vi "IMUBegin.vi"(8 "error in":errorcluster) -> (0 "error out":errorcluster)   [LabVIEW 2014]
uses:
  NavX/roborio/labview/navX-MXP Library/navX-MXP IMU.lvlib
panel:
  out "IMU Opened":bool
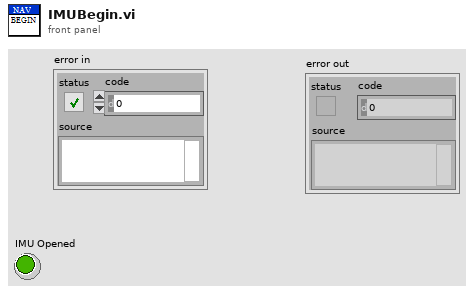
[diagram p1: front panel]
types:
  T1 = typedef "navX-MXP IMU.lvlib/navX Device TypeDef.ctl" = cluster{"navX Interface Protocol":T2, "navX Interface Protocol TypeDefs":cluster{"SPIDevRef":T3, "I2CDevRef":T6}, "navX System Information":cluster{"Board Information":T8, "Status":T9, "Offsets":T13}, "navX Common Information":cluster{"Update Rate (4Hz-60Hz)":T14, "refnum name":string, "error":errorcluster}}
  T2 = typedef "navX-MXP IMU.lvlib/navX Interface Protocol.ctl" = enum16{"SPI", "I2C"}
  T3 = typedef "WPI_SPIDevRef.ctl" = cluster{"DevStatus":errorcluster, "Handle":i32, "Controller":T4, "SPI Bus":T5}
  T4 = typedef "FPGA_TypedefDigitalModule.ctl" = enum16{"Controller 1"}
  T5 = typedef "spi_bus.ctl" = enum16{"SPI On-Board, CS0", "SPI On-Board, CS1", "SPI On-Board, CS2", "SPI On-Board, CS3", "SPI MXP", "Invalid"}
  T6 = typedef "WPI_I2CDevRef.ctl" = cluster{"DevStatus":errorcluster, "Controller":T4, "Device Address":u8, "Handle":i32, "I2C Bus":T7}
  T7 = typedef "i2c_bus.ctl" = enum16{"I2C On-Board", "I2C MXP", "Invalid"}
  T8 = typedef "navX-MXP IMU.lvlib/navX Board Information.ctl" = cluster{"WhoAmI (50 | 0x32)":u8, "Board Revision":u8, "Firmware Major Version":u8, "Firmware Minor Version":u8}
  T9 = typedef "navX-MXP IMU.lvlib/navX Status Data.ctl" = cluster{"Update Rate Hz":u8, "Accelerometer Full-Scale Range":u8, "Gyro Full-Scale Range":u16, "NAVX_OP_STATUS":T10, "NAVX_CAL_STATUS":T11, "NAVX_SELFTEST_STATUS":u8, "NAVX_SENSOR_STATUS":T12}
  T10 = typedef "navX-MXP IMU.lvlib/navX NAVX_OP_STATUS.ctl" = u8
  T11 = typedef "navX-MXP IMU.lvlib/navX NAVX_CAL_STATUS.ctl" = u8
  T12 = typedef "navX-MXP IMU.lvlib/navX NAVX_SENSOR_STATUS.ctl" = cluster{"MOVING":bool, "YAW_STABLE":bool, "MAG_DISTURBANCE":bool, "ALTITUDE_VALID":bool, "SEALEVEL_PRESS_SET":bool, "FUSED_HEADING_VALID":bool}
  T13 = typedef "navX-MXP IMU.lvlib/navX Offsets Data.ctl" = cluster{"Yaw":dbl, "Quat W":dbl, "Quat X":dbl, "Quat Y":dbl, "Quat Z":dbl}
  T14 = typedef "navX-MXP IMU.lvlib/navX Update Rate.ctl" = u8
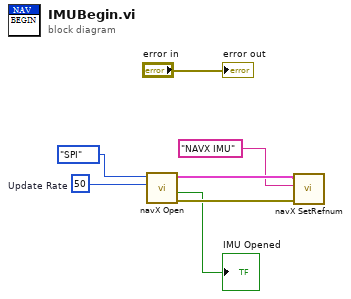
[diagram p0: block diagram]
diagram:
  w7 = 50  # Update Rate
  n1 = call "navX Open.vi"("Update Rate (4Hz-60Hz)"=w7, "navX Interface Protocol"=enum16{"SPI", "I2C"}."SPI") -> ("error out"=w5:errorcluster, "Opened?"=→"IMU Opened":bool, "navX Device TypeDef"=w4:T1)  [unwired: 7 in]
  n2 = call "navX SetRefnum.vi"("error in (no error)"=w5, "refnum name"="NAVX IMU", "navX Device TypeDef"=w4) -> ()  [unwired: 7 in, 2 out]
  "error out" <- "error in"
